vi "Read Configuration Channels.vi"(8 "error in (no error)":errorcluster, 11 "NI-SWITCH Init Parameters in":refnum<class "NI-SWITCH Init Parameters.lvclass">) -> (0 "error out":errorcluster, 2 "Configuration Channels":string[](array[string]), 3 "NI-SWITCH Init Parameters out":refnum<class "NI-SWITCH Init Parameters.lvclass">)   [LabVIEW 2020, in "NI-SWITCH Messaging.lvlib" / "NI-SWITCH Init Parameters.lvclass"]
uses:
  NI-SWITCH Init Parameters.lvclass
  NI-SWITCH Init Parameters.lvclass/NI-SWITCH Init Parameters.ctl
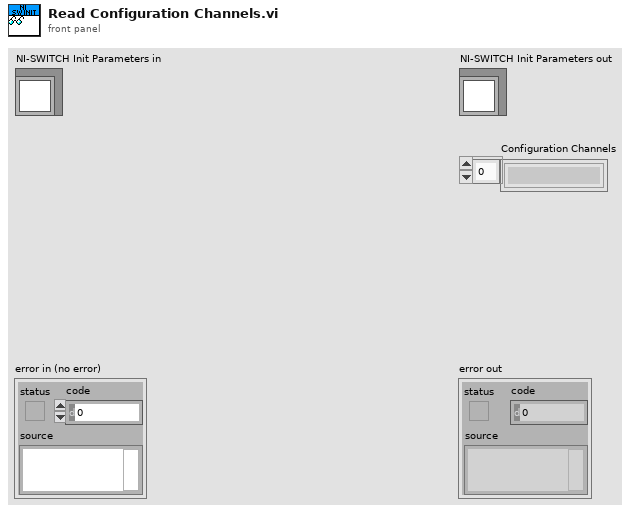
[diagram p1: front panel]
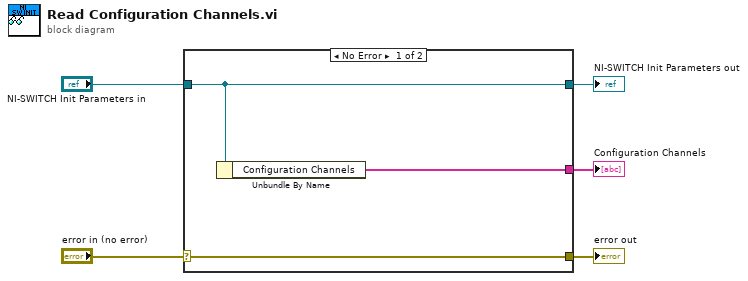
[diagram p0: block diagram]
diagram:
  n1 = case shown="No Error" "error in (no error)" {
    selector: "error in (no error)" -> [w8 w9]
    tunnel: [w8 w9] -> w4
    tunnel: [w7 w10] -> w2
    tunnel: "NI-SWITCH Init Parameters in" -> [w7 w10]
    tunnel: [w6 _] -> w1
    frame No Error {
      n2 = Unbundle By Name(w7) -> ("Configuration Channels"=w6:string[])
    }
    frame Error {
    }
  }
  "error out" <- w4
  "NI-SWITCH Init Parameters out" <- w2
  "Configuration Channels" <- w1
